vi "VIE.Module.Queued Message Handler.dqClass_NotAReference.vi"(1 "reference":T1) -> (0 "not a reference?":bool)   [LabVIEW 2010, in "VIE.Module.Queued Message Handler.QueuedMessageHandler.dqGOOPClass.lvlib"]
doc: "Returns TRUE if dqGOOP object refnum is not a refnum. Otherwise, this function returns FALSE. Use this function to make sure a refnum to a dqGOOP object still resides in system memory and was not closed."
uses:
  VIE.Module.Queued Message Handler.QueuedMessageHandler.dqGOOPClass.lvlib
  VIE.Module.Queued Message Handler.dqClass_ObjectReference.ctl
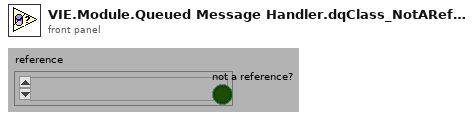
[diagram p1: front panel]
types:
  T1 = typedef "VIE.Module.Queued Message Handler.QueuedMessageHandler.dqGOOPClass.lvlib/VIE.Module.Queued Message Handler.dqClass_ObjectReference.ctl" = refnum<k1>
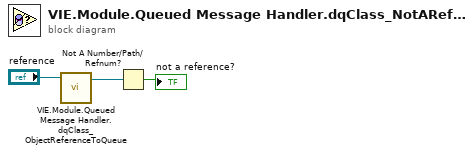
[diagram p0: block diagram]
diagram:
  n1 = call "VIE.Module.Queued Message Handler.dqClass_ObjectReferenceToQueue.vi"("reference"="reference") -> ("queue"=w2:refnum<queue>)  [unwired: 26 in]
  n2 = Not A Number/Path/Refnum?(number/path/refnum=w2) -> (NaN/Path/Refnum?=→"not a reference?":bool)
